vi "VI Tree.vi"   [LabVIEW 2021, in "Agilent N6900 N7900 Series.lvlib"]
doc: "This is the instrument driver for the Agilent N6900 N7900 Series. The VI Tree displays all the user-callable VIs of the instrument driver in an organized table."
uses:
  <instrlib>/Agilent N6900 N7900 Series/Agilent N6900 N7900 Series.lvlib
  <instrlib>/Agilent N6900 N7900 Series/Public/Configure/Arbitrary Waveform/Configure Arbitrary Waveform (Voltage).vi
panel:
  # "(c) 2013-2018 National Instruments Corporation.  ALL RIGHTS RESERVED."
  # "SEE DIAGRAM\nFOR VI TREE."
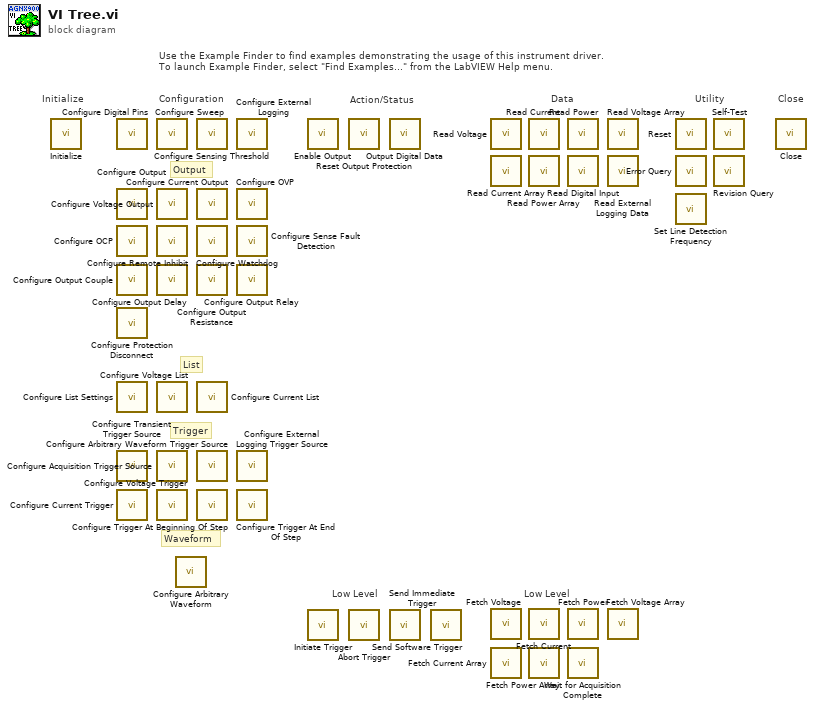
[diagram p0: block diagram]
diagram:
  # "Low Level"
  # "Low Level"
  # "Waveform"
  # "Trigger"
  # "List"
  # "Output"
  # "Use the Example Finder to find examples demonstrating the usage of this instrument driver.\nTo launch Example Finder, select \"Find Examples...\" from the LabVIEW Help menu."
  # "Configuration"
  # "Utility"
  # "Data"
  # "Action/Status"
  # "Close"
  # "Initialize"
  n1 = call <instrlib>:"Initialize.vi"() -> ()  [unwired: 10 in, 2 out]
  n2 = call <instrlib>:"Configure Digital Pins.vi"() -> ()  [unwired: 10 in, 2 out]
  n3 = call <instrlib>:"Configure Output.vi"() -> ()  [unwired: 10 in, 2 out]
  n4 = call <instrlib>:"Configure OCP.vi"() -> ()  [unwired: 10 in, 2 out]
  n5 = call <instrlib>:"Configure Output Couple.vi"() -> ()  [unwired: 10 in, 2 out]
  n6 = call <instrlib>:"Configure Protection Disconnect.vi"() -> ()  [unwired: 10 in, 2 out]
  n7 = call <instrlib>:"Configure List Settings.vi"() -> ()  [unwired: 10 in, 2 out]
  n8 = call <instrlib>:"Configure Transient Trigger Source.vi"() -> ()  [unwired: 10 in, 2 out]
  n9 = call <instrlib>:"Configure Current Trigger.vi"() -> ()  [unwired: 10 in, 2 out]
  n10 = call <instrlib>:"Configure Sweep.vi"() -> ()  [unwired: 10 in, 2 out]
  n11 = call <instrlib>:"Configure Voltage Output.vi"() -> ()  [unwired: 14 in, 2 out]
  n12 = call <instrlib>:"Configure Remote Inhibit.vi"() -> ()  [unwired: 10 in, 2 out]
  n13 = call <instrlib>:"Configure Output Delay.vi"() -> ()  [unwired: 10 in, 2 out]
  n14 = call <instrlib>:"Configure Voltage List.vi"() -> ()  [unwired: 10 in, 2 out]
  n15 = call <instrlib>:"Configure Acquisition Trigger Source.vi"() -> ()  [unwired: 10 in, 2 out]
  n16 = call <instrlib>:"Configure Voltage Trigger.vi"() -> ()  [unwired: 10 in, 2 out]
  n17 = call-poly <instrlib>:"Configure Arbitrary Waveform.vi"() -> ()  [unwired: 10 in, 2 out]
  n18 = call <instrlib>:"Configure Sensing Threshold.vi"() -> ()  [unwired: 10 in, 2 out]
  n19 = call <instrlib>:"Configure Current Output.vi"() -> ()  [unwired: 14 in, 2 out]
  n20 = call <instrlib>:"Configure Watchdog.vi"() -> ()  [unwired: 10 in, 2 out]
  n21 = call <instrlib>:"Configure Output Resistance.vi"() -> ()  [unwired: 10 in, 2 out]
  n22 = call <instrlib>:"Configure Current List.vi"() -> ()  [unwired: 10 in, 2 out]
  n23 = call <instrlib>:"Configure Arbitrary Waveform Trigger Source.vi"() -> ()  [unwired: 10 in, 2 out]
  n24 = call <instrlib>:"Configure Trigger At Beginning Of Step.vi"() -> ()  [unwired: 10 in, 2 out]
  n25 = call <instrlib>:"Configure External Logging.vi"() -> ()  [unwired: 14 in, 2 out]
  n26 = call <instrlib>:"Configure OVP.vi"() -> ()  [unwired: 10 in, 2 out]
  n27 = call <instrlib>:"Configure Sense Fault Detection.vi"() -> ()  [unwired: 10 in, 2 out]
  n28 = call <instrlib>:"Configure Output Relay.vi"() -> ()  [unwired: 10 in, 2 out]
  n29 = call <instrlib>:"Configure External Logging Trigger Source.vi"() -> ()  [unwired: 10 in, 2 out]
  n30 = call <instrlib>:"Configure Trigger At End Of Step.vi"() -> ()  [unwired: 10 in, 2 out]
  n31 = call <instrlib>:"Enable Output.vi"() -> ()  [unwired: 10 in, 2 out]
  n32 = call <instrlib>:"Initiate Trigger.vi"() -> ()  [unwired: 10 in, 2 out]
  n33 = call <instrlib>:"Reset Output Protection.vi"() -> ()  [unwired: 10 in, 2 out]
  n34 = call <instrlib>:"Abort Trigger.vi"() -> ()  [unwired: 10 in, 2 out]
  n35 = call <instrlib>:"Output Digital Data.vi"() -> ()  [unwired: 10 in, 2 out]
  n36 = call <instrlib>:"Send Immediate Trigger.vi"() -> ()  [unwired: 10 in, 2 out]
  n37 = call <instrlib>:"Send Software Trigger.vi"() -> ()  [unwired: 10 in, 2 out]
  n38 = call <instrlib>:"Read Voltage.vi"() -> ()  [unwired: 8 in, 8 out]
  n39 = call <instrlib>:"Read Current Array.vi"() -> ()  [unwired: 9 in, 3 out]
  n40 = call <instrlib>:"Fetch Voltage.vi"() -> ()  [unwired: 8 in, 8 out]
  n41 = call <instrlib>:"Fetch Current Array.vi"() -> ()  [unwired: 9 in, 3 out]
  n42 = call <instrlib>:"Read Current.vi"() -> ()  [unwired: 8 in, 8 out]
  n43 = call <instrlib>:"Read Power Array.vi"() -> ()  [unwired: 9 in, 3 out]
  n44 = call <instrlib>:"Fetch Current.vi"() -> ()  [unwired: 8 in, 8 out]
  n45 = call <instrlib>:"Fetch Power Array.vi"() -> ()  [unwired: 9 in, 3 out]
  n46 = call <instrlib>:"Read Power.vi"() -> ()  [unwired: 9 in, 3 out]
  n47 = call <instrlib>:"Read Digital Input.vi"() -> ()  [unwired: 9 in, 3 out]
  n48 = call <instrlib>:"Fetch Power.vi"() -> ()  [unwired: 9 in, 3 out]
  n49 = call <instrlib>:"Wait for Acquisition Complete.vi"() -> ()  [unwired: 10 in, 2 out]
  n50 = call <instrlib>:"Read Voltage Array.vi"() -> ()  [unwired: 9 in, 3 out]
  n51 = call <instrlib>:"Read External Logging Data.vi"() -> ()  [unwired: 9 in, 3 out]
  n52 = call <instrlib>:"Fetch Voltage Array.vi"() -> ()  [unwired: 9 in, 3 out]
  n53 = call <instrlib>:"Reset.vi"() -> ()  [unwired: 10 in, 2 out]
  n54 = call <instrlib>:"Error Query.vi"() -> ()  [unwired: 8 in, 4 out]
  n55 = call <instrlib>:"Set Line Detection Frequency.vi"() -> ()  [unwired: 10 in, 2 out]
  n56 = call <instrlib>:"Self-Test.vi"() -> ()  [unwired: 8 in, 4 out]
  n57 = call <instrlib>:"Revision Query.vi"() -> ()  [unwired: 8 in, 4 out]
  n58 = call <instrlib>:"Close.vi"() -> ()  [unwired: 11 in, 1 out]
